vi "Setup TestRunner Files.vi"(5 "Interactive (T)":bool=TRUE, 6 "Inspect Recursively (T)":bool=TRUE, 7 "Verbose (F)":bool, 8 "error in (no error)":errorcluster, 9 "Test Report":refnum<class "Test Report.lvclass">, 10 "Paths":path[](array[path]), 11 "Test Runner.Folder":refnum<class "Test Runner.Folder.lvclass">) -> (0 "error out":errorcluster, 3 "Test Runner.Folder out":refnum<class "Test Runner.Folder.lvclass">)   [LabVIEW 2013, in "Caraya.lvlib" / "Test Runner.Folder.lvclass"]
uses:
  Test Runner.Folder.lvclass
  Test Report/Test Report.lvclass
  Test Runner/Test Runner.lvclass/Test Runner.ctl
  Test Runner.Folder.lvclass/Test Runner.Folder.ctl
  Test Runner/Test Runner.lvclass
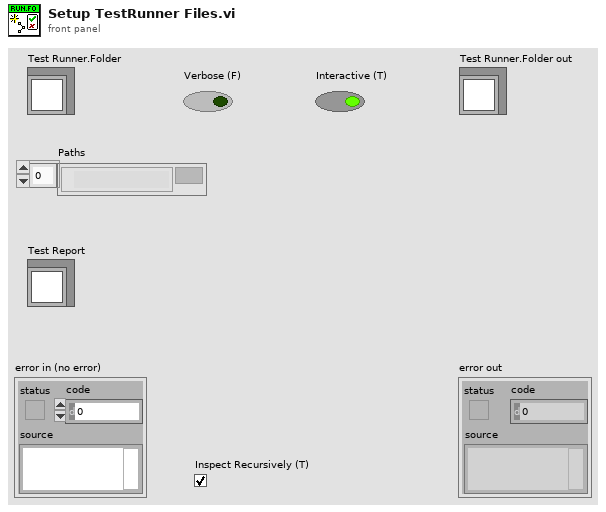
[diagram p1: front panel]
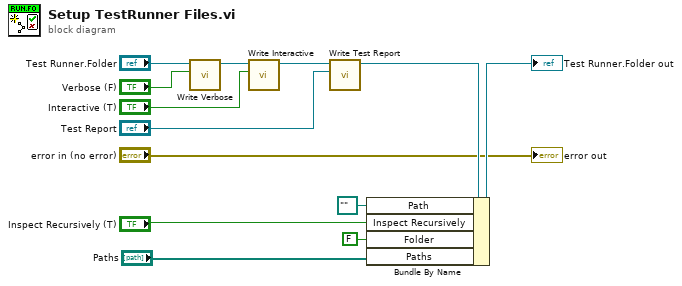
[diagram p0: block diagram]
diagram:
  n1 = call "Write Verbose.vi"("Verbose"="Verbose (F)", "Test Runner in"="Test Runner.Folder") -> ("Test Runner out"=w7:refnum<class "Test Runner.Folder.lvclass">)  [unwired: 9 in]
  n2 = call "Write Interactive.vi"("Interactive"="Interactive (T)", "Test Runner in"=w7) -> ("Test Runner out"=w6:refnum<class "Test Runner.Folder.lvclass">)  [unwired: 9 in]
  n3 = call "Write Test Report.vi"("Test Report"="Test Report", "Test Runner in"=w6) -> ("Test Runner out"=w11:refnum<class "Test Runner.Folder.lvclass">)  [unwired: 9 in]
  n4 = Bundle By Name(cluster=w11, "Path"=path "", "Inspect Recursively"="Inspect Recursively (T)", "Folder"=FALSE, "Paths"="Paths") -> (→"Test Runner.Folder out":refnum<class "Test Runner.Folder.lvclass">)
  "error out" <- "error in (no error)"
